vi "Event-Driven State Machine.vi"() -> ()   [LabVIEW 2020]
uses:
  support/State Machine Data.ctl
  support/States.ctl
  <vilib>/DAQmx/create/channels.llb/DAQmx Create Channel (AO-Voltage-Basic).vi
  <vilib>/DAQmx/configure/timing.llb/DAQmx Timing (Sample Clock).vi
  <vilib>/DAQmx/read.llb/DAQmx Read (Analog 2D DBL NChan NSamp).vi
  <vilib>/Utility/file.llb/Write Delimited Spreadsheet (DBL).vi
  <vilib>/DAQmx/write.llb/DAQmx Write (Analog DBL 1Chan 1Samp).vi
  <vilib>/DAQmx/create/channels.llb/DAQmx Create Channel (AI-Voltage-Basic).vi
panel:
  out "RMS Results Per Channel":dbl[](array[numeric])
  out "Threshold exceeded?":bool
  in  "Acquire":bool
  in  "Samples per channel":i32=100
  in  "Sample Rate":dbl=1000.0
  in  "AI Voltage Channel":tag="PCI-6221/ai0, PCI-6221/ai3"
  in  "AO Voltage Channel":tag="PCI-6221/ai0:1"
  in  "Generate Stimulus":bool
  in  "Threshold (rms)":dbl=1.0
  in  "Clear":bool
  in  "Exit":bool
  out "Graph":dbl[][](graph)
  # "Analysis"
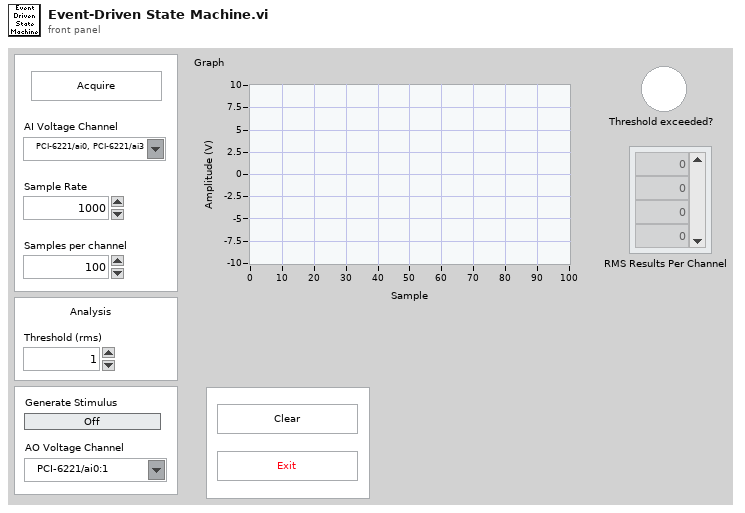
[diagram p1: front panel]
types:
  T1 = typedef "States.ctl" = enum16{"Initialize", "Wait for Event", "Acquire", "Analyze", "Log", "Clear", "Update Stimulus", "Update Graph", "Exit"}
  T2 = typedef "State Machine Data.ctl" = cluster{"Acquisition Data":dbl[][], "Stimulus Value":bool}
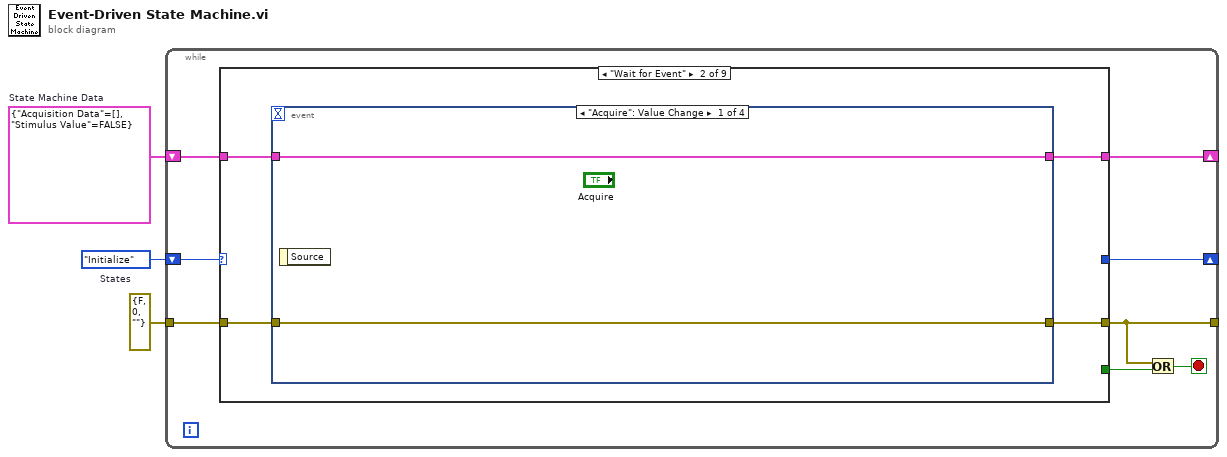
[diagram p0: block diagram]
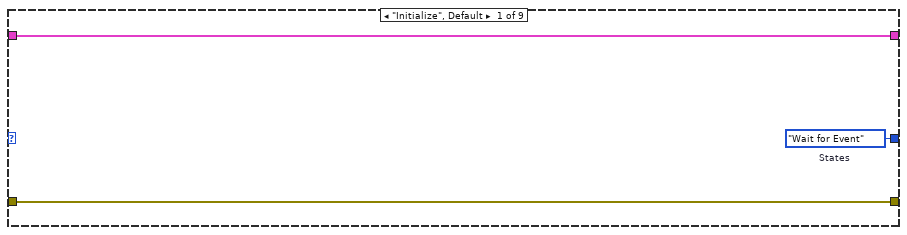
[diagram p2: hidden frame]
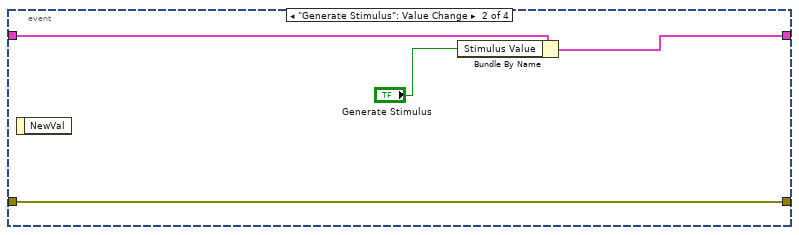
[diagram p3: hidden frame]
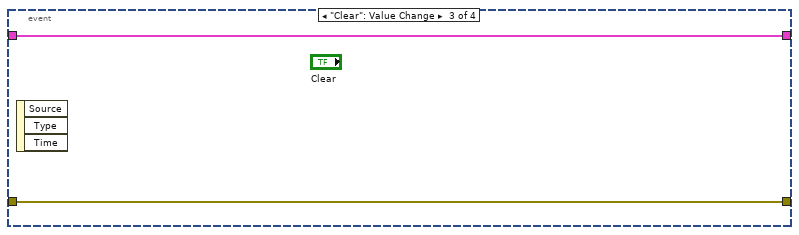
[diagram p4: hidden frame]
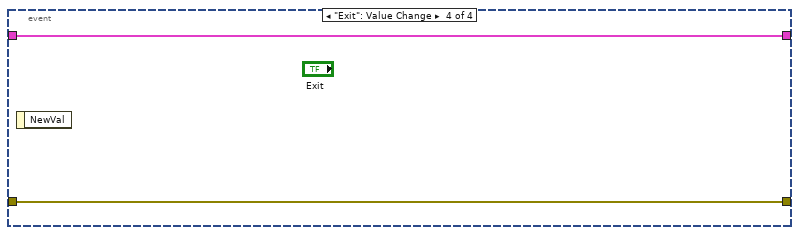
[diagram p5: hidden frame]
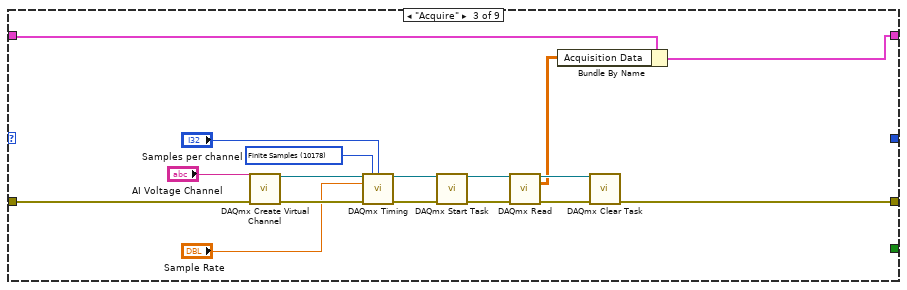
[diagram p6: hidden frame]
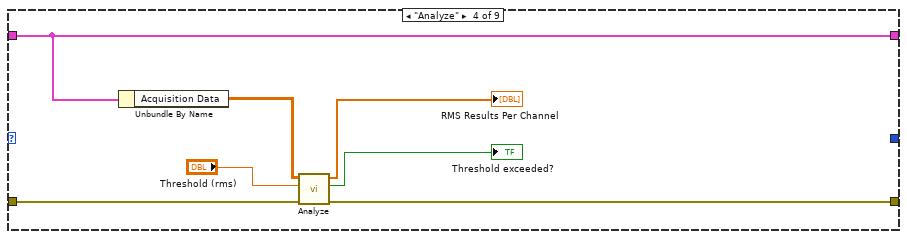
[diagram p7: hidden frame]
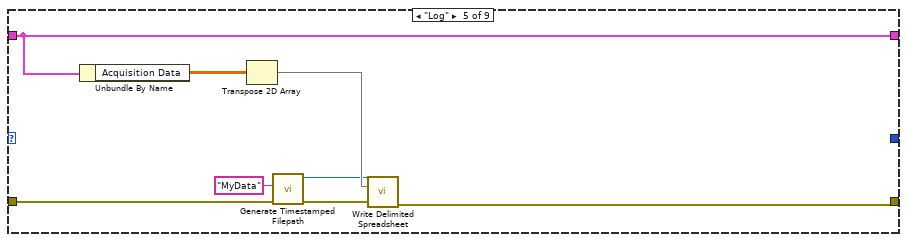
[diagram p8: hidden frame]
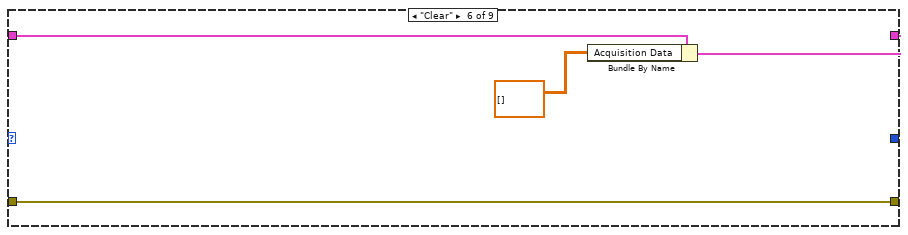
[diagram p9: hidden frame]
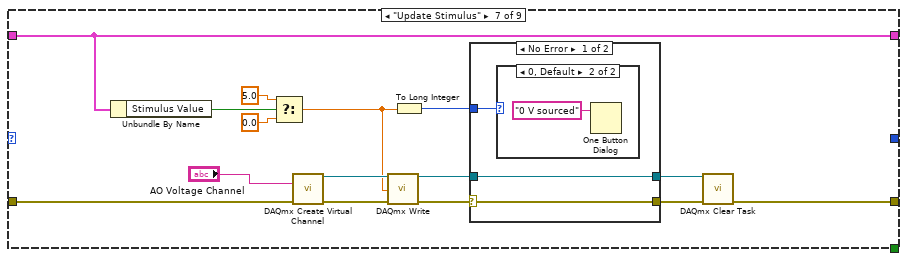
[diagram p10: hidden frame]
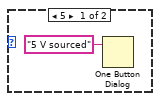
[diagram p11: hidden frame]
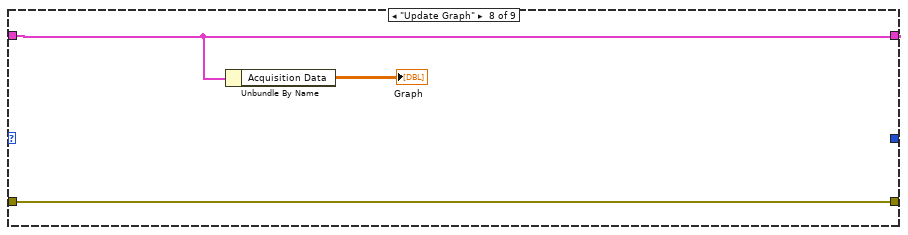
[diagram p13: hidden frame]
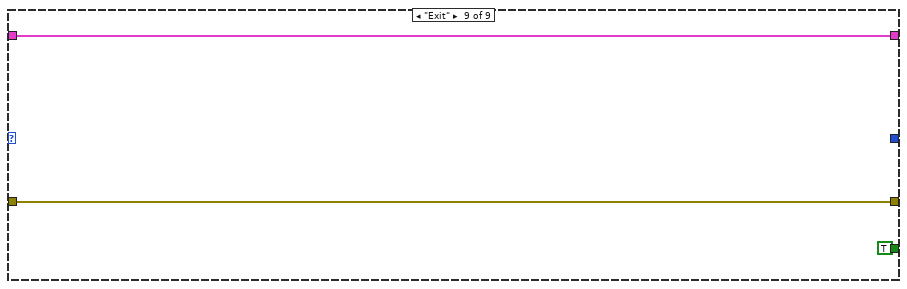
[diagram p14: hidden frame]
diagram:
  w3 = States."Initialize"  # States
  w2 = T2 {"Acquisition Data"=[], "Stimulus Value"=FALSE}  # State Machine Data
  n1 = while {
    shift-right: [w8] -> _
    shift-left: w3 -> [w11]
    shift-right: [w9] -> _
    shift-left: w2 -> [w10]
    tunnel: errorcluster {"status"=FALSE, "code"=0, "source"=""} ("error constant") -> [w7]
    tunnel: [w6] -> _
    stop <- w4 stop-if-true
    n2 = case shown="\"Wait for Event\"" w11 {
      tunnel: w10 -> [w14 w18 w33 w52 w59 w63 w79 w88 w91]
      tunnel: [w14 w17 w31 w52 w59 w61 w79 w88 w91] -> w9
      tunnel: [w13 _ _ _ _ _ _ _ _] -> w8
      tunnel: w7 -> [w12 w16 w45 w49 w57 w64 w72 w89 w92]
      tunnel: [w12 w15 w30 w46 w53 w64 w73 w89 w92] -> w6
      tunnel: [_ _ _ _ _ _ _ _ TRUE] -> w5
      frame "Initialize", Default {
        w13 = States."Wait for Event"  # States
      }
      frame "Wait for Event" {
        n3 = event shown="[0] \"Acquire\": Value Change" {
          selector: _ -> [_ _ _ _]
          dyn-events: _ -> [_ _ _ _]
          timeout: _ -> [_ _ _ _]
          tunnel: w18 -> [w19 w24 w26 w27]
          tunnel: [w19 w23 w26 w27] -> w17
          tunnel: w16 -> [w20 w22 w25 w28]
          tunnel: [w20 w22 w25 w28] -> w15
          event "Acquire": Value Change {
            n4 = event-data() -> ()  [unwired: 1 in, 1 out]
          }
          event "Generate Stimulus": Value Change {
            n5 = event-data() -> ()  [unwired: 1 in, 1 out]
            n6 = Bundle By Name(cluster=w24, "Stimulus Value"="Generate Stimulus") -> (w23:T2)
          }
          event "Clear": Value Change {
            n7 = event-data() -> ()  [unwired: 1 in, 3 out]
          }
          event "Exit": Value Change {
            n8 = event-data() -> ()  [unwired: 1 in, 1 out]
          }
        }
      }
      frame "Acquire" {
        w41 = 10178 items=["Finite Samples"=10178, "Continuous Samples"=10123, "Hardware Timed Single Point"=12522] ("sample mode")
        n9 = call-poly <vilib>:"DAQmx Create Virtual Channel.vi"("physical channels"="AI Voltage Channel", "error in"=w45) -> ("task out"=w42:refnum<k21>, "error out"=w43:errorcluster)  [unwired: 12 in]
        n10 = call-poly <vilib>:"DAQmx Timing.vi"("task/channels in"=w42, "sample mode"=w41, "samples per channel"="Samples per channel", "rate"="Sample Rate", "error in"=w43) -> ("task out"=w39:refnum<k21>, "error out"=w38:errorcluster)  [unwired: 9 in]
        n11 = call <vilib>:"DAQmx Start Task.vi"("task/channels in"=w39, "error in"=w38) -> ("task out"=w37:refnum<k21>, "error out"=w36:errorcluster)  [unwired: 12 in]
        n12 = call-poly <vilib>:"DAQmx Read.vi"("task/channels in"=w37, "error in"=w36) -> ("task out"=w35:refnum<k21>, "data"=w32:dbl[][], "error out"=w34:errorcluster)  [unwired: 11 in]
        n13 = Bundle By Name(cluster=w33, "Acquisition Data"=w32) -> (w31:T2)
        n14 = call <vilib>:"DAQmx Clear Task.vi"("task in"=w35, "error in"=w34) -> ("error out"=w30:errorcluster)  [unwired: 13 in]
      }
      frame "Analyze" {
        n15 = Unbundle By Name(w52) -> ("Acquisition Data"=w51:dbl[][])
        n16 = call "Analyze.vi"("error in (no error)"=w49, "Threshold (rms)"="Threshold (rms)", "N-Channel Data (2D DBL)"=w51) -> ("error out"=w46:errorcluster, "Threshold Exceeded?"=→"Threshold exceeded?":bool, "N-Channel RMS Results"=→"RMS Results Per Channel":dbl[])  [unwired: 5 in, 1 out]
      }
      frame "Log" {
        n17 = Unbundle By Name(w59) -> ("Acquisition Data"=w60:dbl[][])
        n18 = Transpose 2D Array(2D array=w60) -> (transposed array=w56:dbl[][])
        n19 = call "Generate Timestamped Filepath.vi"("Error In"=w57, "appended filename"="MyData") -> ("Error Out"=w54:errorcluster, "timestamped relative filepath"=w55:path)  [unwired: 8 in]
        n20 = call-poly <vilib>:"Write Delimited Spreadsheet.vi"("file path (dialog if empty)"=w55, "2D data"=w56, "error in (no error)"=w54) -> ("error out"=w53:errorcluster)  [unwired: 11 in, 1 out]
      }
      frame "Clear" {
        n21 = Bundle By Name(cluster=w63, "Acquisition Data"=dbl[][] []) -> (w61:T2)
      }
      frame "Update Stimulus" {
        n22 = Unbundle By Name(w79) -> ("Stimulus Value"=w78:bool)
        n23 = Select(t=5.0, s=w78, f=0.0) -> (s? t:f=w70:dbl)
        n24 = call-poly <vilib>:"DAQmx Create Virtual Channel.vi"("physical channels"="AO Voltage Channel", "error in"=w72) -> ("task out"=w75:refnum<k21>, "error out"=w74:errorcluster)  [unwired: 12 in]
        n25 = call-poly <vilib>:"DAQmx Write.vi"("task/channels in"=w75, "data"=w70, "error in"=w74) -> ("task out"=w66:refnum<k21>, "error out"=w68:errorcluster)  [unwired: 10 in, 1 out]
        n26 = To Long Integer(number=w70) -> (32bit integer=w69:i32)
        n27 = case shown="No Error" w68 {
          selector: w68 -> [w81 w85]
          tunnel: w69 -> [w82 _]
          tunnel: [w81 w85] -> w67
          tunnel: w66 -> [w80 w86]
          tunnel: [w80 w86] -> w65
          frame No Error {
            n28 = case shown="0, Default" w82 {
              frame 5 {
                n29 = One Button Dialog(message="5 V sourced") -> ()  [unwired: 1 in, 1 out]
              }
              frame 0, Default {
                n30 = One Button Dialog(message="0 V sourced") -> ()  [unwired: 1 in, 1 out]
              }
            }
          }
          frame Error {
          }
        }
        n31 = call <vilib>:"DAQmx Clear Task.vi"("task in"=w65, "error in"=w67) -> ("error out"=w73:errorcluster)  [unwired: 13 in]
      }
      frame "Update Graph" {
        n32 = Unbundle By Name(w88) -> ("Acquisition Data"=→"Graph":dbl[][])
      }
      frame "Exit" {
      }
    }
    n33 = Or(x=w6, y=w5) -> (x .or. y?=w4:bool)
  }
